vi "校准信息读取.vi"(8 "Error in":errorcluster caption="Error in (no error)", 11 "Slave ID":u8=1) -> (0 "error out":errorcluster, 3 "校准信息读取":T1 {"校准类型" items=["单点校准"=1, "两点校准"=2, "三点校准"=3]})   [LabVIEW 2016, in "斯坦道原位多参数.lvlib"]
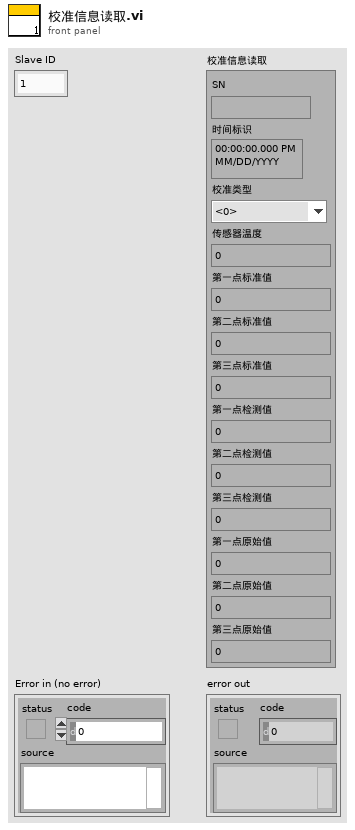
[diagram p1: front panel]
types:
  T1 = cluster{"SN":string, "时间标识":timestamp, "校准类型":u16, "传感器温度":sgl, "第一点标准值":sgl, "第二点标准值":sgl, "第三点标准值":sgl, "第一点检测值":sgl, "第二点检测值":sgl, "第三点检测值":sgl, "第一点原始值":sgl, "第二点原始值":sgl, "第三点原始值":sgl}
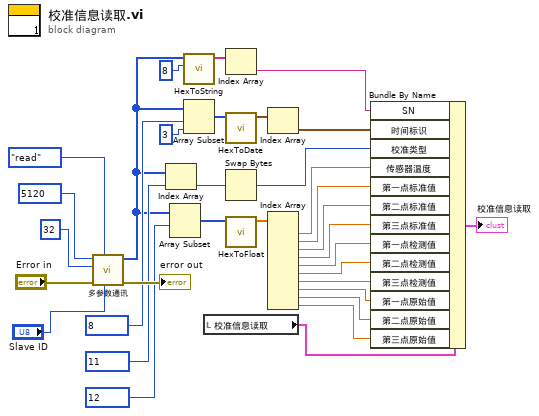
[diagram p0: block diagram]
diagram:
  n1 = call "多参数通讯.vi"("Slave ID"="Slave ID", "STEP"=enum16{"open", "read", "write", "close"}."read", "Error in"="Error in", "quantity"=u16 32, "starting address"=u16 5120) -> ("error out"=→"error out":errorcluster, "Registers"=w23:u16[])  [unwired: 4 in, 1 out]
  n2 = Index Array(array=w23, index=u16 11 ("starting address")) -> (element=w3:u16)
  n3 = Array Subset(array=w23, index=u16 12 ("starting address")) -> (w21:u16[])  [unwired: 1 in]
  n4 = call "HexToString.vi"("字符个数"=8, "数组"=w23) -> ("STRING"=w18:string[])  [unwired: 9 in]
  n5 = Array Subset(array=w23, index=u16 8 ("starting address"), length=3 ("长度")) -> (w25:u16[])
  n6 = local read "校准信息读取"() -> (w20:T1)
  n7 = Index Array(array=w18) -> (element=w17:string)  [unwired: 1 in]
  n8 = call "HexToDate.vi"("数组"=w25) -> ("DATE"=w16:timestamp[])  [unwired: 10 in]
  n9 = Swap Bytes(anything=w3) -> (byte swapped=w2:u16)
  n10 = call "HexToFloat.vi"("数组"=w21) -> ("FLOAT"=w14:sgl[])  [unwired: 10 in]
  n11 = Index Array(array=w16) -> (element=w15:timestamp)  [unwired: 1 in]
  n12 = Index Array(array=w14) -> (element #1=w13:sgl, element #2=w12:sgl, element #3=w11:sgl, element #4=w10:sgl, element #5=w9:sgl, element #6=w8:sgl, element #7=w7:sgl, element #8=w6:sgl, element #9=w5:sgl, element #10=w4:sgl)  [unwired: 10 in]
  n13 = Bundle By Name(cluster=w20, "SN"=w17, "时间标识"=w15, "校准类型"=w2, "传感器温度"=w13, "第一点标准值"=w12, "第二点标准值"=w11, "第三点标准值"=w10, "第一点检测值"=w9, "第二点检测值"=w8, "第三点检测值"=w7, "第一点原始值"=w6, "第二点原始值"=w5, "第三点原始值"=w4) -> (→"校准信息读取":T1)
